vi "Double Histogram (G) v2.vi"(0 "Array":dbl[](array[numeric]), 1 "Project Outside Values onto Boundaries (F)":bool, 2 "Max Histogram Size (10^5)":i32=100000, 5 "Bin Size (Sturge's Rule)":dbl, 7 "Min (Array Min)":dbl=nan, 9 "Max (Array Max)":dbl=nan, 11 "Filter NaN, +/- Inf (F)":bool, 12 "Normalized (F)":bool, 13 "Aligned Bins (F)":bool, 14 "Bin Location (Left)":T2) -> (4 "Axis":dbl[](array[numeric]), 6 "Histogram":dbl[](array[numeric]), 15 "Array Statistics":T1)   [LabVIEW 2019]
doc: "If Min or Max are not provided, they are set to the Array Min or Max.\nIf one of the bounds is infinite, the histogram is not computed.\nIf Bin Size is not provided, or has a bogus value (< or = 0, Inf), Sturge's rule is used."
uses:
  Histogram Bin Position.ctl
  Array Statistics.ctl
  929807a6-00f9-4258-af09-20dfd637e3ca.vi/021b2fa1-60c1-478e-a41e-827a580c90b5.vi
  <vilib>/Analysis/NI_AALBase.lvlib
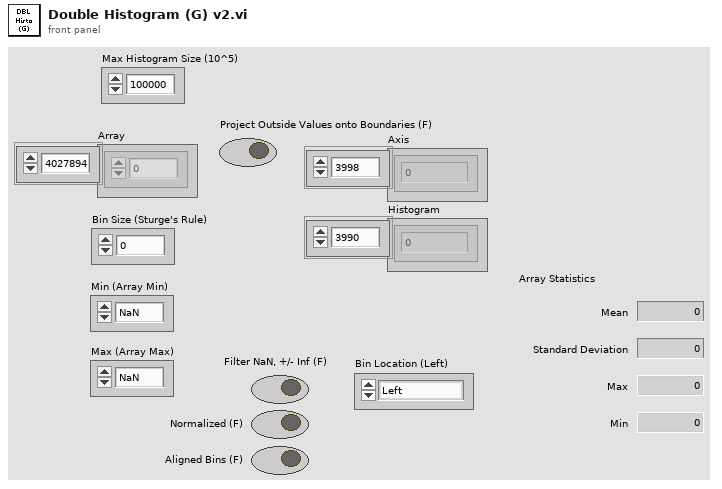
[diagram p1: front panel]
types:
  T1 = typedef "Array Statistics.ctl" = cluster{"Mean":dbl, "Standard Deviation":dbl, "Max":dbl, "Min":dbl}
  T2 = typedef "Histogram Bin Position.ctl" = enum16{"Left", "Center", "Right"}
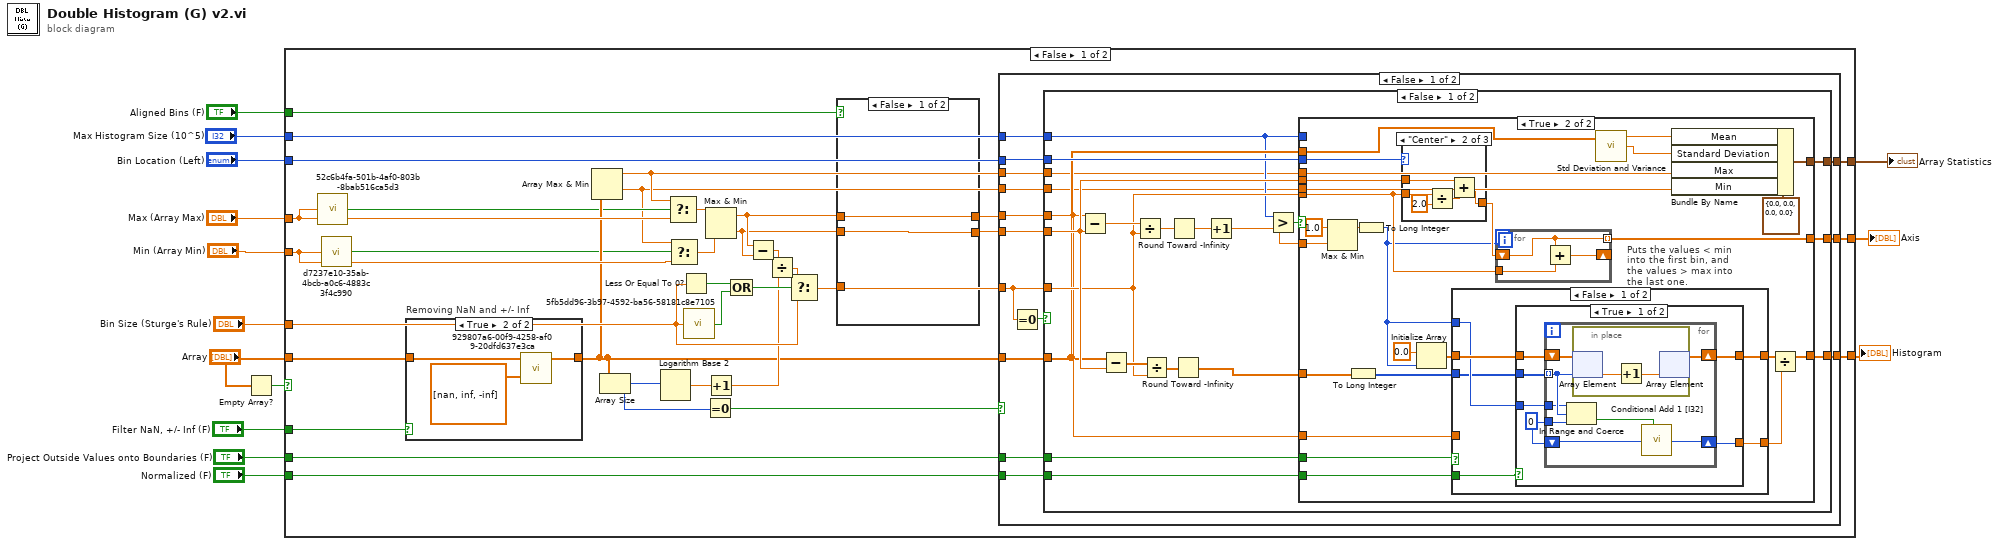
[diagram p0: block diagram]
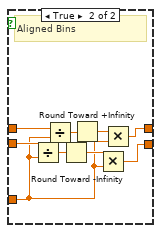
[diagram p2: hidden frame]
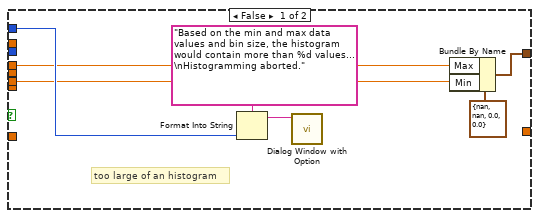
[diagram p4: hidden frame]
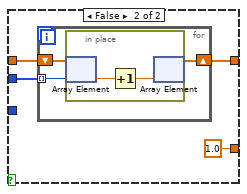
[diagram p5: hidden frame]
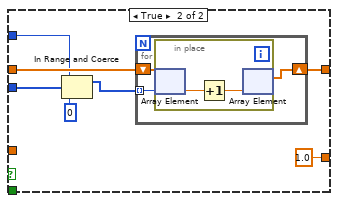
[diagram p6: hidden frame]
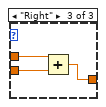
[diagram p8: hidden frame]
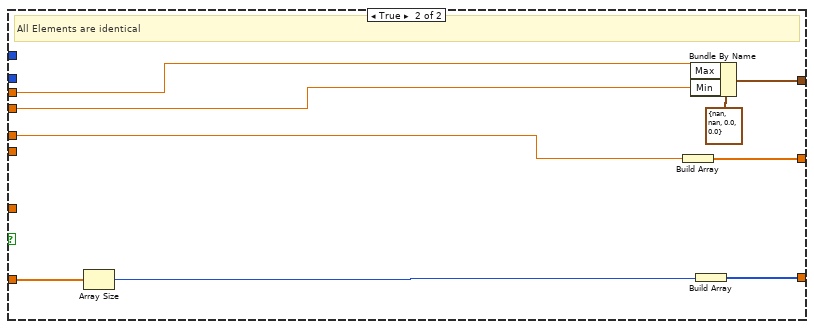
[diagram p9: hidden frame]
diagram:
  n1 = Empty Array?(array="Array") -> (empty?=w4:bool)
  n2 = case shown="False" w4 {
    tunnel: [w48 _] -> w14
    tunnel: [w47 _] -> w13
    tunnel: "Min (Array Min)" -> [w46 _]
    tunnel: "Max (Array Max)" -> [w45 _]
    tunnel: "Bin Size (Sturge's Rule)" -> [w38 _]
    tunnel: "Bin Location (Left)" -> [w35 _]
    tunnel: "Project Outside Values onto Boundaries (F)" -> [w34 _]
    tunnel: "Filter NaN, +/- Inf (F)" -> [w32 _]
    tunnel: "Max Histogram Size (10^5)" -> [w26 _]
    tunnel: "Array" -> [w25 _]
    tunnel: [w24 _] -> w3
    tunnel: "Normalized (F)" -> [w23 _]
    tunnel: "Aligned Bins (F)" -> [w22 _]
    frame False {
      n3 = call "52c6b4fa-501b-4af0-803b-8bab516ca5d3.vi"("Number"=w45) -> ("Is NaN or Inf?"=w30:bool)  [unwired: 8 in]
      n4 = call "d7237e10-35ab-4bcb-a0c6-4883c3f4c990.vi"("Number"=w46) -> ("Is NaN or Inf?"=w31:bool)  [unwired: 8 in]
      n5 = case "Removing NaN and +/- Inf" shown="True" w32 {
        tunnel: w25 -> [w60 w63]
        tunnel: [w60 w62] -> w33
        frame False {
        }
        frame True {
          n6 = call "929807a6-00f9-4258-af09-20dfd637e3ca.vi"("Element(s) to Remove"=dbl[] [nan, inf, -inf], "Input Array"=w63) -> ("Output Array"=w62:dbl[])  [unwired: 1 out]
        }
      }
      n7 = Array Max & Min(array=w33) -> (max value=w20:dbl, min value=w19:dbl)  [unwired: 2 out]
      n8 = Array Size(array=w33) -> (size(s)=w29:i32)
      n9 = Logarithm Base 2(1:w29) -> (0:w39:dbl)
      n10 = Select(t=w20, s=w30, f=w45) -> (s? t:f=w43:dbl)
      n11 = Select(t=w19, s=w31, f=w46) -> (s? t:f=w44:dbl)
      n12 = Less Or Equal To 0?(x=w38) -> (x <= 0?=w42:bool)
      n13 = call "5fb5dd96-3b97-4592-ba56-58181c8e7105.vi"("Number"=w38) -> ("Is NaN or Inf?"=w41:bool)  [unwired: 8 in]
      n14 = Equal To 0?(x=w29) -> (x = 0?=w28:bool)
      n15 = Max & Min(x=w43, y=w44) -> (max(x,y)=w18:dbl, min(x,y)=w17:dbl)
      n16 = Increment(x=w39) -> (x+1=w36:dbl)
      n17 = Compound Arithmetic op=OR(w42, w41) -> (w40:bool)
      n18 = Subtract(x=w18, y=w17) -> (x-y=w37:dbl)
      n19 = Divide(x=w37, y=w36) -> (x/y=w27:dbl)
      n20 = Select(t=w27, s=w40, f=w38) -> (s? t:f=w21:dbl)
      n21 = case shown="False" w22 {
        tunnel: w21 -> [_ w52]
        tunnel: w18 -> [w50 w55]
        tunnel: w17 -> [w49 w59]
        tunnel: [w50 w51] -> w16
        tunnel: [w49 w56] -> w15
        frame False {
        }
        frame True {
          # "Aligned Bins"
          n22 = Divide(x=w59, y=w52) -> (x/y=w58:dbl)
          n23 = Divide(x=w55, y=w52) -> (x/y=w54:dbl)
          n24 = Round Toward -Infinity(1:w58) -> (0:w57:dbl)
          n25 = Round Toward +Infinity(x=w54) -> (ceil(x): smallest int >= x=w53:dbl)
          n26 = Multiply(x=w57, y=w52) -> (x*y=w56:dbl)
          n27 = Multiply(x=w53, y=w52) -> (x*y=w51:dbl)
        }
      }
      n28 = case shown="False" w28 {
        tunnel: [w77 _] -> w48
        tunnel: w21 -> [w70 _]
        tunnel: [w76 _] -> w47
        tunnel: w33 -> [w71 _]
        tunnel: w16 -> [w72 _]
        tunnel: w15 -> [w74 _]
        tunnel: w35 -> [w75 _]
        tunnel: w34 -> [w73 _]
        tunnel: w26 -> [w68 _]
        tunnel: [w67 _] -> w24
        tunnel: w23 -> [w66 _]
        tunnel: w20 -> [w65 _]
        tunnel: w19 -> [w64 _]
        frame False {
          n29 = Equal To 0?(x=w70) -> (x = 0?=w69:bool)
          n30 = case shown="False" w69 {
            tunnel: [w97 w195] -> w77
            tunnel: [w94 w192] -> w76
            tunnel: w75 -> [w93 _]
            tunnel: w74 -> [w92 _]
            tunnel: w70 -> [w91 _]
            tunnel: w73 -> [w89 _]
            tunnel: w72 -> [w88 w191]
            tunnel: w71 -> [w87 w194]
            tunnel: w68 -> [w86 _]
            tunnel: [w83 w190] -> w67
            tunnel: w66 -> [w82 _]
            tunnel: w65 -> [w81 w188]
            tunnel: w64 -> [w80 w187]
            frame False {
              n31 = Subtract(x=w88, y=w92) -> (x-y=w98:dbl)
              n32 = Subtract(x=w87, y=w92) -> (x-y=w96:dbl[])
              n33 = Divide(x=w98, y=w91) -> (x/y=w90:dbl)
              n34 = Divide(x=w96, y=w91) -> (x/y=w95:dbl[])
              n35 = Round Toward -Infinity(1:w90) -> (0:w78:dbl)
              n36 = Round Toward -Infinity(1:w95) -> (0:w79:dbl[])
              n37 = Increment(x=w78) -> (x+1=w85:dbl)
              n38 = Greater?(x=w86, y=w85) -> (0:w84:bool)
              n39 = case shown="True" w84 {
                tunnel: [_ w131] -> w97
                tunnel: w79 -> [_ w129]
                tunnel: [_ w114] -> w94
                tunnel: w93 -> [_ w127]
                tunnel: w92 -> [_ w126]
                tunnel: w91 -> [_ w124]
                tunnel: w89 -> [_ w123]
                tunnel: w88 -> [_ w122]
                tunnel: w87 -> [_ w106]
                tunnel: w85 -> [_ w121]
                tunnel: w86 -> [w103 _]
                tunnel: [w99 w117] -> w83
                tunnel: w82 -> [_ w110]
                tunnel: w81 -> [w102 w109]
                tunnel: w80 -> [w101 w108]
                frame False {
                  # "too large of an histogram"
                  n40 = Format Into String(format string="Based on the min and max data values and bin size, the histogram would contain more than %d values...\nHistogramming aborted." ("message"), w103) -> (resulting string=w105:string)  [unwired: 2 in, 1 out]
                  n41 = call "Dialog Window with Option.vi"("Message"=w105) -> ()  [unwired: 8 in, 3 out]
                  n42 = Bundle By Name(cluster=T1 {"Mean"=nan, "Standard Deviation"=nan, "Max"=0.0, "Min"=0.0} ("Array Statistics"), "Max"=w102, "Min"=w101) -> (w99:T1)
                }
                frame True {
                  n43 = Max & Min(x=1.0, y=w121) -> (max(x,y)=w113:dbl)  [unwired: 1 out]
                  n44 = To Long Integer(number=w129) -> (32bit integer=w111:i32[])
                  n45 = To Long Integer(number=w113) -> (32bit integer=w112:i32)
                  n46 = case shown="\"Center\"" w127 {
                    tunnel: w126 -> [w175 w178 w183]
                    tunnel: [w175 w176 w182] -> w125
                    tunnel: w124 -> [_ w180 w181]
                    frame "Left", Default {
                    }
                    frame "Center" {
                      n47 = Divide(x=w180, y=2.0) -> (x/y=w177:dbl)
                      n48 = Add(x=w178, y=w177) -> (x+y=w176:dbl)
                    }
                    frame "Right" {
                      n49 = Add(x=w183, y=w181) -> (x+y=w182:dbl)
                    }
                  }
                  n50 = Initialize Array(0.0 ("element"), w112) -> (w128:dbl[])
                  n51 = case "Puts the values < min into the first bin, and the values > max into the last one." shown="False" w123 {
                    tunnel: w111 -> [w132 w166]
                    tunnel: w128 -> [w137 w169]
                    tunnel: [w136 w168] -> w116
                    tunnel: w122 -> [_ _]
                    tunnel: w112 -> [w135 w165]
                    tunnel: [w134 1.0 ("lower limit")] -> w115
                    tunnel: w110 -> [w133 _]
                    frame False {
                      n52 = case shown="True" w133 {
                        tunnel: w137 -> [w143 w157]
                        tunnel: [w142 w156] -> w136
                        tunnel: w132 -> [w141 w155]
                        tunnel: w135 -> [w140 _]
                        tunnel: [w138 1.0 ("lower limit")] -> w134
                        frame True {
                          w139 = 0 ("lower limit")
                          n53 = for {
                            tunnel: w141 -> [w149] mode=indexing
                            shift-right: [w150] -> w142
                            shift-left: w143 -> [w151]
                            tunnel: w139 -> [w148]
                            tunnel: w140 -> [w147]
                            shift-right: [w144] -> w138
                            shift-left: w139 -> [w145]
                            n54 = In Range and Coerce(upper limit=w147, x=w149, lower limit=w148) -> (In Range?=w146:bool)  [unwired: 1 out]
                            n55 = in-place {
                              n56 = in-place-array #1(w151, w149) -> (w153:dbl)
                              n57 = Increment(x=w153) -> (x+1=w152:dbl)
                              n58 = in-place-array #1(w152) -> (w150:dbl[])  [unwired: 1 out]
                            }
                            n59 = call "Conditional Add 1 [I32].vi"("Condition"=w146, "x"=w145) -> ("x (+1)"=w144:i32)  [unwired: 7 in]
                          }
                        }
                        frame False {
                          n60 = for {
                            tunnel: w155 -> [w158] mode=indexing
                            shift-right: [w159] -> w156
                            shift-left: w157 -> [w160]
                            n61 = in-place {
                              n62 = in-place-array #2(w160, w158) -> (w162:dbl)
                              n63 = Increment(x=w162) -> (x+1=w161:dbl)
                              n64 = in-place-array #2(w161) -> (w159:dbl[])  [unwired: 1 out]
                            }
                          }
                        }
                      }
                    }
                    frame True {
                      n65 = In Range and Coerce(upper limit=w165, x=w166, lower limit=0) -> (coerced(x)=w164:i32[])  [unwired: 1 out]
                      n66 = for {
                        shift-right: [w171] -> w168
                        shift-left: w169 -> [w172]
                        tunnel: w164 -> [w170] mode=indexing
                        n67 = in-place {
                          n68 = in-place-array #3(w172, w170) -> (w174:dbl)
                          n69 = Increment(x=w174) -> (x+1=w173:dbl)
                          n70 = in-place-array #3(w173) -> (w171:dbl[])  [unwired: 1 out]
                        }
                      }
                    }
                  }
                  n71 = for {
                    N: w112 -> [_]
                    shift-right: [w185] -> _
                    shift-left: w125 -> [w184]
                    tunnel: w124 -> [w186]
                    tunnel: [w184] -> w131 mode=indexing
                    n72 = Add(x=w184, y=w186) -> (x+y=w185:dbl)
                  }
                  n73 = call <vilib>:"Std Deviation and Variance.vi"("X"=w106) -> ("mean"=w119:dbl, "standard deviation"=w118:dbl)  [unwired: 1 in, 1 out]
                  n74 = Bundle By Name(cluster=T1 {"Mean"=0.0, "Standard Deviation"=0.0, "Max"=0.0, "Min"=0.0} ("Array Statistics"), "Mean"=w119, "Standard Deviation"=w118, "Max"=w109, "Min"=w108) -> (w117:T1)
                  n75 = Divide(x=w116, y=w115) -> (x/y=w114:dbl[])
                }
              }
            }
            frame True {
              # "All Elements are identical"
              n76 = Array Size(array=w194) -> (size(s)=w193:i32)
              n77 = Build Array(w191) -> (w195:dbl[])
              n78 = Bundle By Name(cluster=T1 {"Mean"=nan, "Standard Deviation"=nan, "Max"=0.0, "Min"=0.0} ("Array Statistics"), "Max"=w188, "Min"=w187) -> (w190:T1)
              n79 = Build Array(w193) -> (w192:i32[])
            }
          }
        }
        frame True {
          # "no valid elements or empty array"
        }
      }
    }
    frame True {
    }
  }
  "Histogram" <- w13
  "Axis" <- w14
  "Array Statistics" <- w3
